vi "Check Trigger.vi"(6 "Values":dbl[](array[numeric]), 8 "error in (no error)":errorcluster, 11 "TriggerDelayControl in":refnum<class "TriggerDelayControl.lvclass">) -> (0 "error out":errorcluster, 2 "Triggered":bool, 3 "TriggerDelayControl out":refnum<class "TriggerDelayControl.lvclass">)   [LabVIEW 2020, in "VolatusControl.lvlib" / "TriggerDelayControl.lvclass"]
uses:
  TriggerDelayControl.lvclass
  TriggerDelayControl.lvclass/TriggerDelayControl.ctl
  lv-vecto/Vecto/Channel/Channel.lvclass
  lv-vecto/Vecto/StringChannel/StringChannel.lvclass
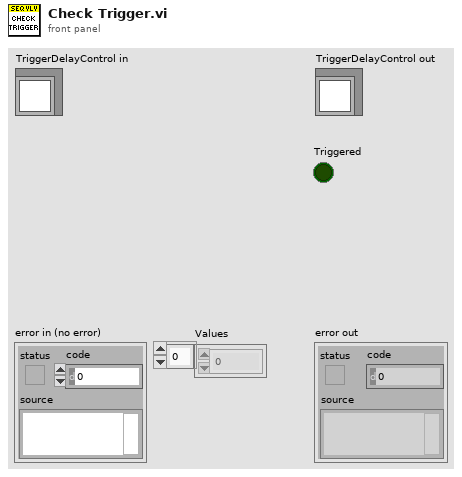
[diagram p1: front panel]
types:
  T1 = typedef "VolatusControl.lvlib/TriggerDelayControl.lvclass/Channel Type.ctl" = enum16{"Double", "String"}
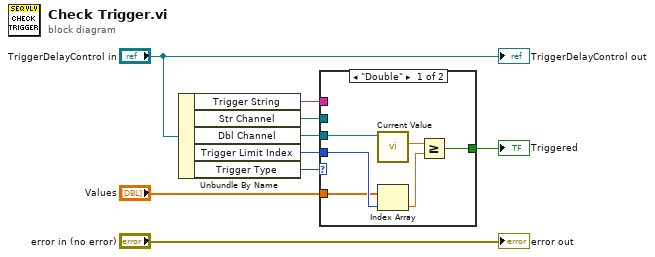
[diagram p0: block diagram]
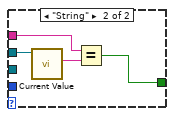
[diagram p2: hidden frame]
diagram:
  n1 = Unbundle By Name("TriggerDelayControl in") -> ("Trigger String"=w2:string, "Str Channel"=w3:refnum<class "StringChannel.lvclass">, "Dbl Channel"=w7:refnum<class "Channel.lvclass">, "Trigger Limit Index"=w8:i32, "Trigger Type"=w4:T1)
  n2 = case shown="\"Double\"" w4 {
    tunnel: w8 -> [w15 _]
    tunnel: w7 -> [w14 _]
    tunnel: "Values" -> [w11 _]
    tunnel: w3 -> [_ w19]
    tunnel: w2 -> [_ w17]
    tunnel: [w10 w16] -> w1
    frame "Double" {
      n3 = call "Current Value.vi"("Channel in"=w14) -> ("Scaled"=w13:dbl)  [unwired: 6 in, 4 out]
      n4 = Index Array(array=w11, index=w15) -> (element=w12:dbl)
      n5 = Greater Or Equal?(x=w13, y=w12) -> (x >= y?=w10:bool)
    }
    frame "String" {
      n6 = call "Current Value.vi"("StringChannel in"=w19) -> ("String"=w18:string)  [unwired: 7 in, 3 out]
      n7 = Equal?(x=w17, y=w18) -> (x = y?=w16:bool)
    }
  }
  "Triggered" <- w1
  "error out" <- "error in (no error)"
  "TriggerDelayControl out" <- "TriggerDelayControl in"
